vi "Query Test Results.vi"(8 "error IO":errorcluster, 11 "VISA resource name":refnum<visa-resource-name>) -> (0 "error Out":errorcluster, 2 "Results":enum16{"NONE", "FAIL", "PASS", "ALL"}(ring), 3 "VISA resource Out":refnum<visa-resource-name>)   [LabVIEW 2020, in "eec EST 300.lvlib"]
doc: "STR?\nReturns the Test Results setting. There are 4 options:\n0=NONE,\n1=FAIL, \n2=PASS, \n3=ALL\nSelect PASS to save the results of the steps that passed. Select FAIL to save the results of the steps that failed. Select ALL to save all the test results. Selecting NONE will not save any results to the internal memory."
uses:
  <instrlib>/eec EST 300/eec EST 300.lvlib
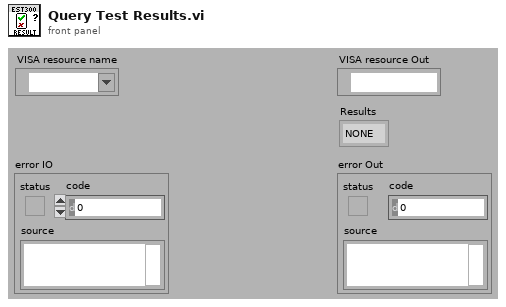
[diagram p1: front panel]
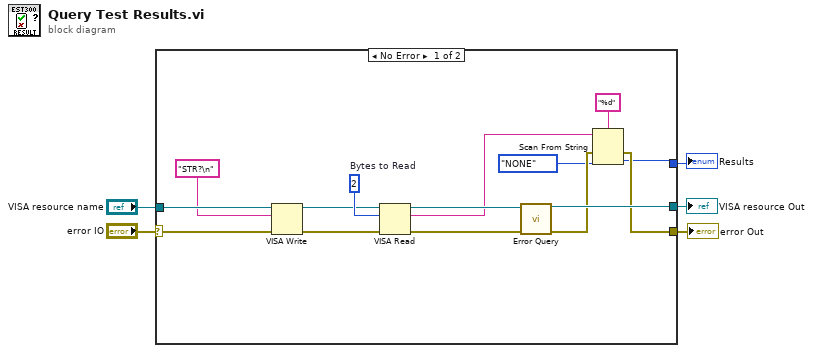
[diagram p0: block diagram]
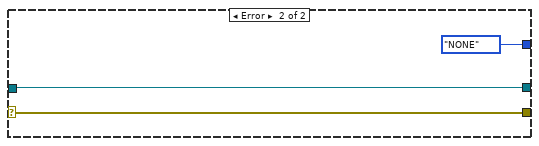
[diagram p2: hidden frame]
diagram:
  n1 = case shown="No Error" "error IO" {
    selector: "error IO" -> [w20 w23]
    tunnel: [w9 w23] -> w2
    tunnel: [w18 w22] -> w3
    tunnel: "VISA resource name" -> [w19 w22]
    tunnel: [w6 enum16{"NONE", "FAIL", "PASS", "ALL"}."NONE" ("Results Display")] -> w1
    frame No Error {
      w14 = u32 2  # Bytes to Read
      n2 = VISA Write(VISA resource name=w19, write buffer="STR?\n" ("Command to Send (empty)"), error in (no error)=w20) -> (VISA resource name out=w13:refnum<visa-resource-name>, error out=w12:errorcluster)  [unwired: 1 out]
      n3 = VISA Read(VISA resource name=w13, byte count=w14, error in (no error)=w12) -> (VISA resource name out=w16:refnum<visa-resource-name>, read buffer=w8:string, error out=w15:errorcluster)  [unwired: 1 out]
      n4 = call <instrlib>:"Error Query.vi"("VISA resource name"=w16, "error in (no error)"=w15) -> ("VISA resource name out"=w18:refnum<visa-resource-name>, "error out"=w10:errorcluster)  [unwired: 10 in, 2 out]
      n5 = Scan From String(format string="%d", input string=w8, error in=w10, default 1=enum16{"NONE", "FAIL", "PASS", "ALL"}."NONE" ("Results Display")) -> (error out=w9:errorcluster, output 1=w6:enum16{"NONE", "FAIL", "PASS", "ALL"})  [unwired: 1 in, 2 out]
    }
    frame Error {
    }
  }
  "VISA resource Out" <- w3
  "error Out" <- w2
  "Results" <- w1
